vi "PointInPolys.vi"(10 "Point2D":T1, 11 "Polys":T2[](array[typedef])) -> (3 "Outside":bool)   [LabVIEW 2014]
uses:
  TypeDefs/Poly2DwSlope.ctl
  TypeDefs/Point2DwSlope.ctl
  <vilib>/Analysis/geometry.llb/Point in Polygon (Scalar).vi
  <vilib>/Analysis/NI_AAL_Geometry.lvlib
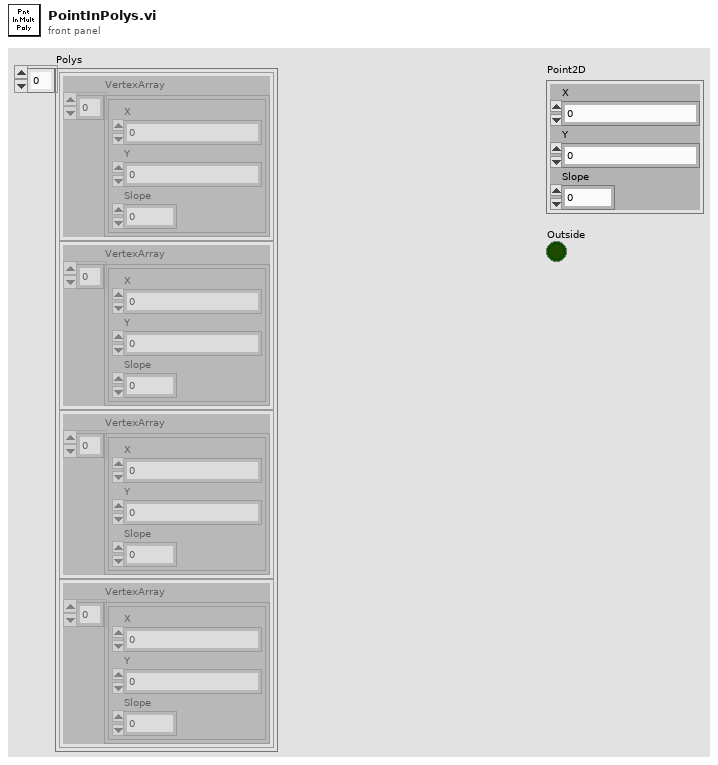
[diagram p1: front panel]
types:
  T1 = typedef "Point2DwSlope.ctl" = cluster{"X":sgl, "Y":sgl, "Slope":dbl}
  T2 = typedef "Poly2DwSlope.ctl" = cluster{"VertexArray":T1[]}
  T3 = typedef "NI_AAL_Geometry.lvlib/Point in Polygon Position.ctl" = u16
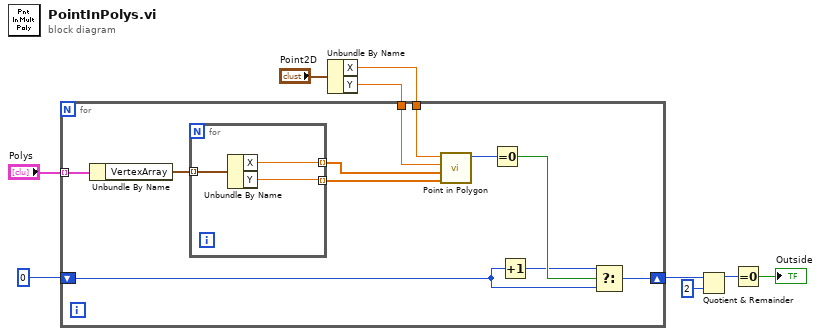
[diagram p0: block diagram]
diagram:
  n1 = Unbundle By Name("Point2D") -> ("X"=w8:sgl, "Y"=w7:sgl)
  n2 = for {
    tunnel: "Polys" -> [w20] mode=indexing
    tunnel: w8 -> [w16]
    tunnel: w7 -> [w15]
    shift-right: [w12] -> w4
    shift-left: 0 -> [w10]
    n3 = Unbundle By Name(w20) -> ("VertexArray"=w19:T1[])
    n4 = for {
      tunnel: w19 -> [w23] mode=indexing
      tunnel: [w22] -> w17 mode=indexing
      tunnel: [w21] -> w18 mode=indexing
      n5 = Unbundle By Name(w23) -> ("X"=w22:sgl, "Y"=w21:sgl)
    }
    n6 = call-poly <vilib>:"Point in Polygon.vi"("Polygon Y"=w18, "Polygon X"=w17, "y"=w15, "x"=w16) -> ("position"=w14:T3)  [unwired: 6 in, 1 out]
    n7 = Equal To 0?(x=w14) -> (x = 0?=w13:bool)
    n8 = Increment(x=w10) -> (x+1=w11:i32)
    n9 = Select(t=w11, s=w13, f=w10) -> (s? t:f=w12:i32)
  }
  n10 = Quotient & Remainder(x=w4, y=2) -> (x-y*floor(x/y)=w2:i32)  [unwired: 1 out]
  n11 = Equal To 0?(x=w2) -> (x = 0?=→"Outside":bool)
